vi "ElectdSet.vi"(8 "Group #":u8, 9 "Amplitude":sgl=-1.0, 10 "Index":u8=15, 11 "Electd Panel in":refnum<vi>) -> (3 "Electd Panel out":refnum<vi>)   [LabVIEW 2012, in "StimulCtrls.lvlib"]
uses:
  StimulCtrls.lvlib
  ElectdTerminal.ctl
panel:
  out "String":string
  in  "T 0":T1 caption="T #"
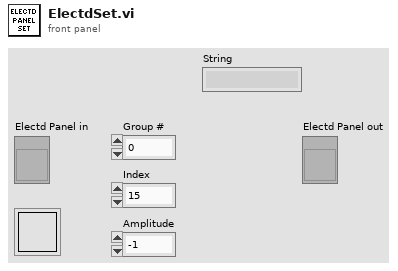
[diagram p1: front panel]
types:
  T1 = typedef "StimulCtrls.lvlib/ElectdTerminal.ctl" = u8
  T2 = enum8{"Enabled", "Disabled", "Disabled and Grayed Out"}
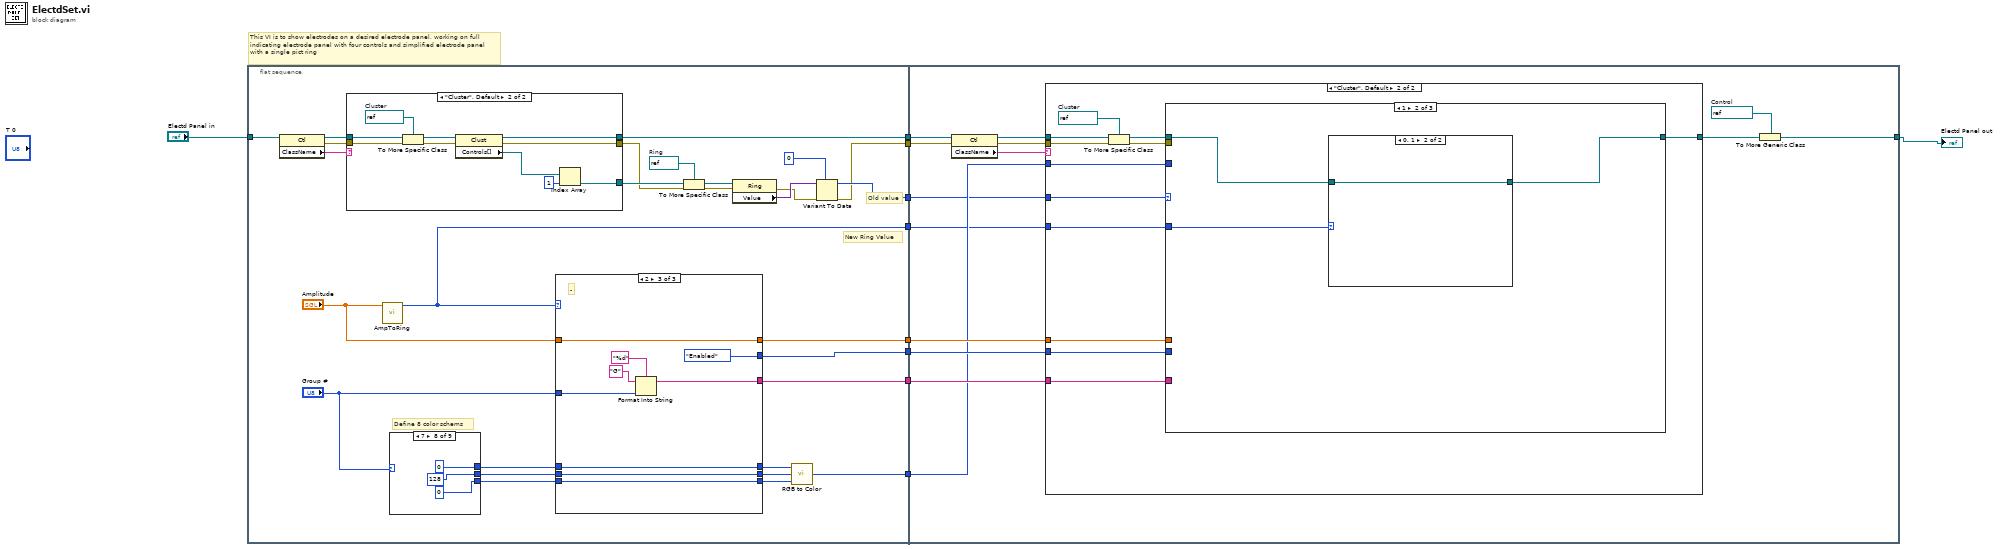
[diagram p0: block diagram]
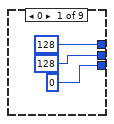
[diagram p3: hidden frame]
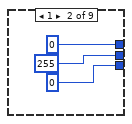
[diagram p4: hidden frame]
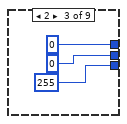
[diagram p5: hidden frame]
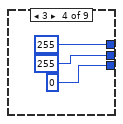
[diagram p6: hidden frame]
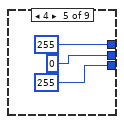
[diagram p7: hidden frame]
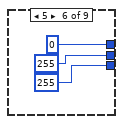
[diagram p8: hidden frame]
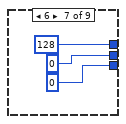
[diagram p9: hidden frame]
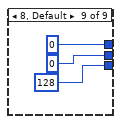
[diagram p10: hidden frame]
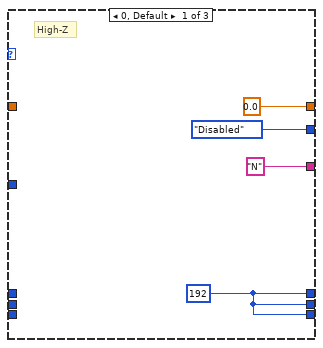
[diagram p11: hidden frame]
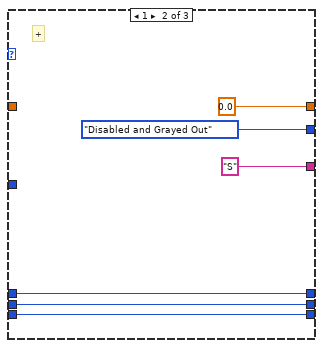
[diagram p12: hidden frame]
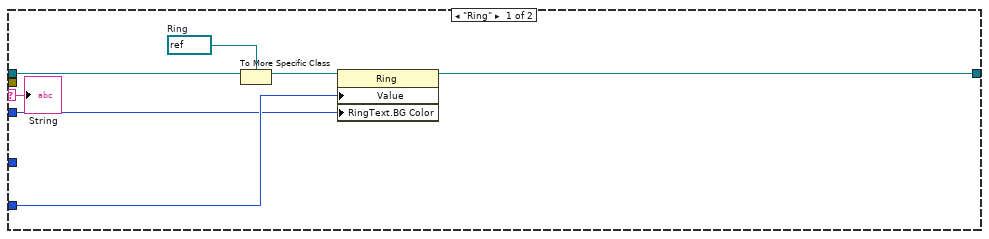
[diagram p13: hidden frame]
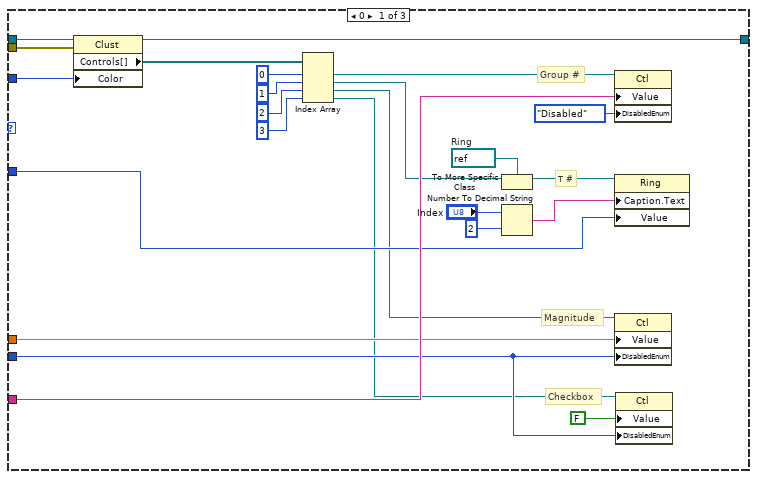
[diagram p14: hidden frame]
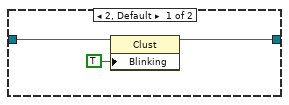
[diagram p15: hidden frame]
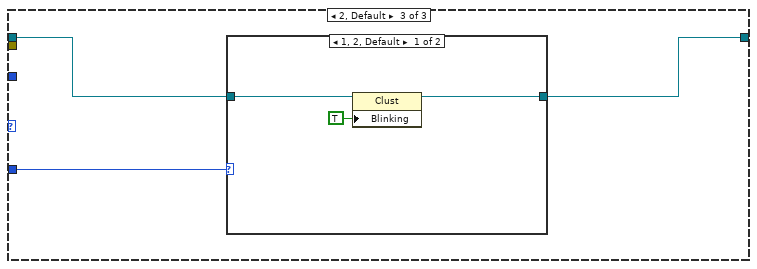
[diagram p16: hidden frame]
diagram:
  # "This VI is to show electrodes on a desired electrode panel, working on full indicating electrode panel with four controls and simplified electrode panel with a single pict ring"
  n1 = flat-sequence {
    tunnel: [w34] -> w10
    tunnel: [w33] -> w9
    tunnel: [w32] -> w8
    tunnel: [w31] -> w7
    tunnel: [w28] -> w6
    tunnel: "Electd Panel in" -> [w20]
    tunnel: [w17] -> w5
    tunnel: [w25] -> w4
    tunnel: [w13] -> w1
    tunnel: w10 -> [w106]
    tunnel: w9 -> [w109]
    tunnel: w8 -> [w107]
    tunnel: w7 -> [w108]
    tunnel: w6 -> [w105]
    tunnel: [w99] -> w3
    tunnel: w5 -> [w103]
    tunnel: w4 -> [w102]
    tunnel: w1 -> [w96]
    frame #0 {
      w18 = refnum<vi> refnum  # Ring
      # "Define 8 color schems"
      # "New Ring Value"
      # "Old value"
      n2 = property class="Ctl"(reference=w20) -> (error out=w11:errorcluster, "ClassName"=w19:string)  [unwired: 1 in, 1 out]
      n3 = case shown="\"Cluster\", Default" w19 {
        tunnel: [w39 w49] -> w29
        tunnel: [w39 w46] -> w28
        tunnel: w20 -> [w39 w45]
        tunnel: [w38 w41] -> w12
        tunnel: w11 -> [w38 w40]
        frame "Ring" {
        }
        frame "Cluster", Default {
          w42 = refnum<vi> refnum  # Cluster
          n4 = To More Specific Class(target class=w42, reference=w45, error in=w40) -> (specific class reference=w44:refnum<vi>, error out=w43:errorcluster)
          n5 = property class="Clust"(reference=w44, error in=w43) -> (reference out=w46:refnum<vi>, error out=w41:errorcluster, "Controls[]"=w47:refnum<vi>[])
          n6 = Index Array(array=w47, index=1) -> (element=w49:refnum<vi>)
        }
      }
      n7 = call "AmpToRing.vi"("Amplitude"="Amplitude") -> ("Ring Value"=w25:u8)  [unwired: 10 in]
      n8 = case shown="7" "Group #" {
        tunnel: [u32 128 ("Color") u32 0 ("Color") u32 0 ("Color") u32 255 ("Color") u32 255 ("Color") u32 0 ("Color") u32 128 ("Color") u32 0 ("Color") u32 0 ("Color")] -> w23
        tunnel: [u32 128 ("Color") u32 255 ("Color") u32 0 ("Color") u32 255 ("Color") u32 0 ("Color") u32 255 ("Color") u32 0 ("Color") u32 128 ("Color") u32 0 ("Color")] -> w22
        tunnel: [u32 0 ("Color") u32 0 ("Color") u32 255 ("Color") u32 0 ("Color") u32 255 ("Color") u32 255 ("Color") u32 0 ("Color") u32 0 ("Color") u32 128 ("Color")] -> w21
        frame 0 {
        }
        frame 1 {
        }
        frame 2 {
        }
        frame 3 {
        }
        frame 4 {
        }
        frame 5 {
        }
        frame 6 {
        }
        frame 7 {
        }
        frame 8, Default {
        }
      }
      n9 = case shown="2" w25 {
        tunnel: ["N" ("Group #") "S" ("Group #") w93] -> w33
        tunnel: [T2."Disabled" ("Disabled") T2."Disabled and Grayed Out" ("Disabled") T2."Enabled" ("Disabled")] -> w31
        tunnel: [w77 w83 w89] -> w35
        tunnel: [w77 w82 w88] -> w36
        tunnel: [w77 w81 w87] -> w37
        tunnel: [sgl 0.0 ("Magnitude") sgl 0.0 ("Magnitude") w94] -> w32
        tunnel: "Amplitude" -> [_ _ w94]
        tunnel: "Group #" -> [_ _ w90]
        tunnel: w23 -> [_ w83 w89]
        tunnel: w22 -> [_ w82 w88]
        tunnel: w21 -> [_ w81 w87]
        frame 0, Default {
          w77 = u32 192 ("Color")
          # "High-Z"
        }
        frame 1 {
          # "+"
        }
        frame 2 {
          # "-"
          n10 = Format Into String(format string="%d", initial string="G", w90) -> (resulting string=w93:string)  [unwired: 1 in, 1 out]
        }
      }
      n11 = To More Specific Class(target class=w18, reference=w29, error in=w12) -> (specific class reference=w30:refnum<vi>, error out=w15:errorcluster)
      n12 = property class="Ring"(reference=w30, error in=w15) -> (error out=w14:errorcluster, "Value"=w26:variant)  [unwired: 1 out]
      n13 = call <vilib>:"RGB to Color.vi"("B"=w37, "G"=w36, "R"=w35) -> ("Color"=w34:u32)
      n14 = Variant To Data(error in=w14, type=0, Variant=w26) -> (data=w17:i32, error out=w13:errorcluster)
    }
    frame #1 {
      w98 = refnum<vi> refnum  # Control
      n15 = property class="Ctl"(reference=w105, error in=w96) -> (reference out=w101:refnum<vi>, error out=w97:errorcluster, "ClassName"=w100:string)
      n16 = case shown="\"Cluster\", Default" w100 {
        selector: w100 -> [w110 _]
        tunnel: w109 -> [_ w128]
        tunnel: w108 -> [_ w127]
        tunnel: w107 -> [_ w126]
        tunnel: w106 -> [w111 w125]
        tunnel: [w113 w124] -> w104
        tunnel: w103 -> [_ w123]
        tunnel: w102 -> [w112 w122]
        tunnel: w101 -> [w116 w121]
        tunnel: w97 -> [_ w118]
        frame "Ring" {
          w115 = refnum<vi> refnum  # Ring
          n17 = To More Specific Class(target class=w115, reference=w116) -> (specific class reference=w114:refnum<vi>)  [unwired: 1 in, 1 out]
          n18 = property class="Ring"(reference=w114, "Value"=w112, "RingText.BG Color"=w111) -> (reference out=w113:refnum<vi>)  [unwired: 1 in, 1 out]
          "String" <- w110
        }
        frame "Cluster", Default {
          w119 = refnum<vi> refnum  # Cluster
          n19 = To More Specific Class(target class=w119, reference=w121, error in=w118) -> (specific class reference=w120:refnum<vi>, error out=w117:errorcluster)
          n20 = case shown="1" w123 {
            tunnel: w128 -> [w152 _ _]
            tunnel: w127 -> [w136 _ _]
            tunnel: w126 -> [w139 _ _]
            tunnel: w125 -> [w135 _ _]
            tunnel: w120 -> [w143 w154 w161]
            tunnel: [w142 w153 w160] -> w124
            tunnel: w122 -> [w141 w155 w162]
            tunnel: w117 -> [w129 _ _]
            frame 0 {
              w144 = refnum<vi> refnum  # Ring
              # "Checkbox"
              # "Group #"
              # "Magnitude"
              # "T #"
              n21 = property class="Clust"(reference=w143, error in=w129, "Color"=w135) -> (reference out=w142:refnum<vi>, "Controls[]"=w134:refnum<vi>[])  [unwired: 1 out]
              n22 = Index Array(array=w134, index #1=0 ("index"), index #2=1 ("index"), index #3=2 ("index"), index #4=3 ("index")) -> (element #1=w133:refnum<vi>, element #2=w132:refnum<vi>, element #3=w131:refnum<vi>, element #4=w130:refnum<vi>)
              n23 = To More Specific Class(target class=w144, reference=w132) -> (specific class reference=w145:refnum<vi>)  [unwired: 1 in, 1 out]
              n24 = Number To Decimal String(number="Index", width (-)=i16 2) -> (decimal integer string=w151:string)
              n25 = property class="Ctl"(reference=w133, "Value"=w152, "DisabledEnum"=T2."Disabled" ("Disabled")) -> ()  [unwired: 1 in, 2 out]
              n26 = property class="Ring"(reference=w145, "Caption.Text"=w151, "Value"=w141) -> ()  [unwired: 1 in, 2 out]
              n27 = property class="Ctl"(reference=w131, "Value"=w139, "DisabledEnum"=w136) -> ()  [unwired: 1 in, 2 out]
              n28 = property class="Ctl"(reference=w130, "Value"=FALSE, "DisabledEnum"=w136) -> ()  [unwired: 1 in, 2 out]
            }
            frame 1 {
              n29 = case shown="0, 1" w155 {
                tunnel: w154 -> [w158 w159]
                tunnel: [w156 w159] -> w153
                frame 2, Default {
                  n30 = property class="Clust"(reference=w158, "Blinking"=TRUE) -> (reference out=w156:refnum<vi>)  [unwired: 1 in, 1 out]
                }
                frame 0, 1 {
                }
              }
            }
            frame 2, Default {
              n31 = case shown="1, 2, Default" w162 {
                tunnel: w161 -> [w164 w166]
                tunnel: [w163 w166] -> w160
                frame 1, 2, Default {
                  n32 = property class="Clust"(reference=w164, "Blinking"=TRUE) -> (reference out=w163:refnum<vi>)  [unwired: 1 in, 1 out]
                }
                frame 0 {
                }
              }
            }
          }
        }
      }
      n33 = To More Generic Class(target class=w98, reference=w104) -> (generic class reference=w99:refnum<vi>)
    }
  }
  "Electd Panel out" <- w3
